vi "New Vision Update from JSON.vi"(2 "error in":errorcluster, 3 "JSON string":string, 4 "Current Time (ms)":i32) -> (0 "error out":errorcluster, 1 "Vision Update":T1)   [LabVIEW 2016]
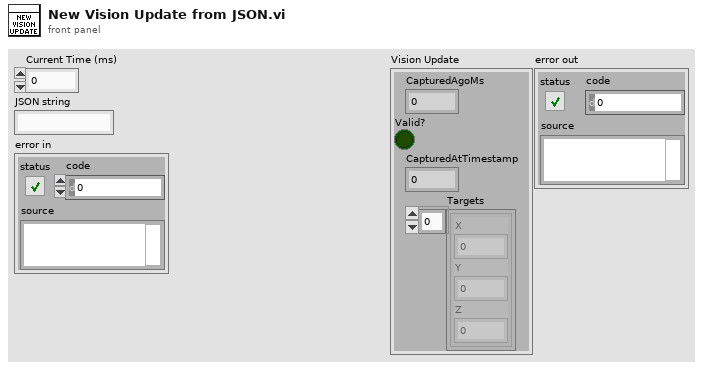
[diagram p1: front panel]
types:
  T1 = cluster{"CapturedAgoMs":i32, "Valid?":bool, "CapturedAtTimestamp":dbl, "Targets":cluster{"X":dbl, "Y":dbl, "Z":dbl}[]}
  T2 = cluster{"CapturedAgoMs":i32, "Targets":cluster{"X":dbl, "Y":dbl, "Z":dbl}[]}
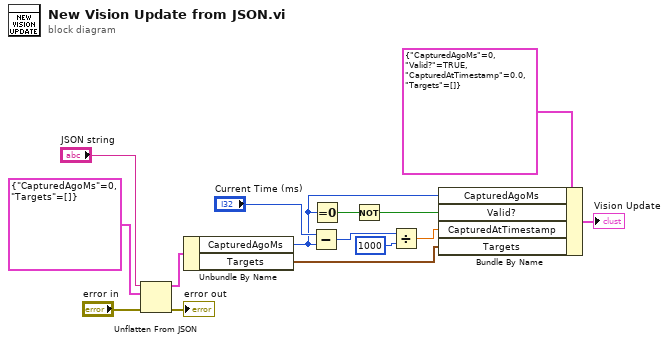
[diagram p0: block diagram]
diagram:
  n1 = Unflatten From JSON(JSON string="JSON string", type and defaults=T2 {"CapturedAgoMs"=0, "Targets"=[]}, error in (no error)="error in") -> (value=w13:T2, error out=→"error out":errorcluster)  [unwired: 4 in]
  n2 = Unbundle By Name(w13) -> ("CapturedAgoMs"=w4:i32, "Targets"=w5:cluster{"X":dbl, "Y":dbl, "Z":dbl}[])
  n3 = Subtract(x="Current Time (ms)", y=w4) -> (x-y=w9:i32)
  n4 = Equal To 0?(x=w4) -> (x = 0?=w11:bool)
  n5 = Not(x=w11) -> (.not. x?=w7:bool)
  n6 = Divide(x=w9, y=1000) -> (x/y=w6:dbl)
  n7 = Bundle By Name(cluster=T1 {"CapturedAgoMs"=0, "Valid?"=TRUE, "CapturedAtTimestamp"=0.0, "Targets"=[]}, "CapturedAgoMs"=w4, "Valid?"=w7, "CapturedAtTimestamp"=w6, "Targets"=w5) -> (→"Vision Update":T1)
